vi "GEA2 Commands Dryer CMD.vi"() -> (2 "CMD Array":u8[](array[numeric])=[115, 0] format="%02x")   [LabVIEW 2016]
doc: "Given the command array, this VI will look up the associated Hex numaric and output that value"
panel:
  in  "Commands":cluster{"String":string, "CMD Array":u8[]}[](array[cluster])=[{"String"="CMD_Eval_Mode_Entry_CC1", "CMD Array"=[112, 1]}, {"String"="CMD_Eval_Mode_Entry_CC2", "CMD Array"=[112, 2]}, {"String"="CMD_Eval_Mode_Continue", "CMD Array"=[113]}, {"String"="CMD_Send_DIAG_Info", "CMD Array"=[114]}, {"String"="CMD_Enable_Debug_Log ", "CMD Array"=[115, 1]}, {"String"="CMD_Disable_Debug_Log ", "CMD Array"=[115, 0]}, {"String"="CMD_Send_Log_Data", "CMD Array"=[116]}, {"String"="CMD_Stop", "CMD Array"=[118]}, {"String"="RQST_Version", "CMD Array"=[1]}] {"CMD Array" format="%02x"}
  out "Data Array":string[][](array[string])=[["CMD_Eval_Mode_Entry_CC1", "0x70", "0x01"], ["CMD_Eval_Mode_Entry_CC2", "0x70", "0x02"], ["CMD_Eval_Mode_Continue", "0x71", "N/A"], ["CMD_Send_DIAG_Info", "0x72", "N/A"], ["CMD_Enable_Debug_Log ", "0x73", "0x01"], ["CMD_Disable_Debug_Log ", "0x73", "0x00"], ["CMD_Send_Log_Data", "0x74", "N/A"]]
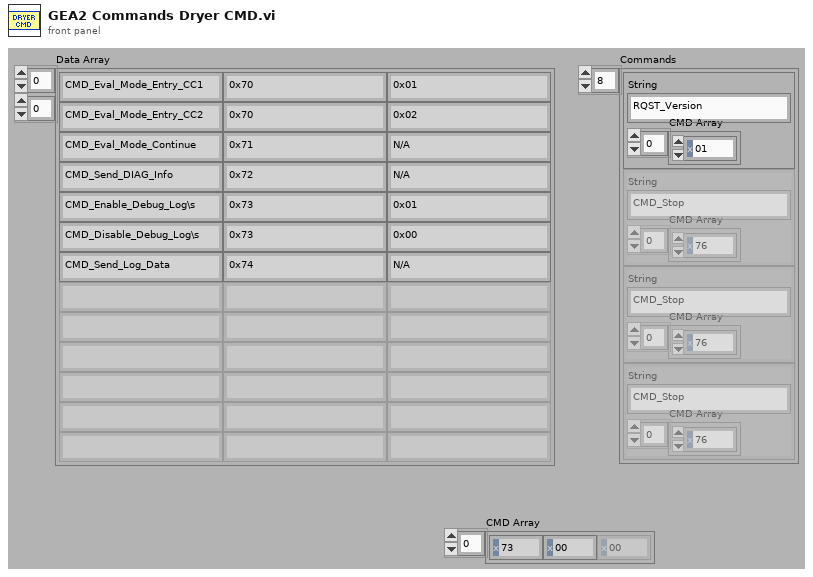
[diagram p1: front panel]
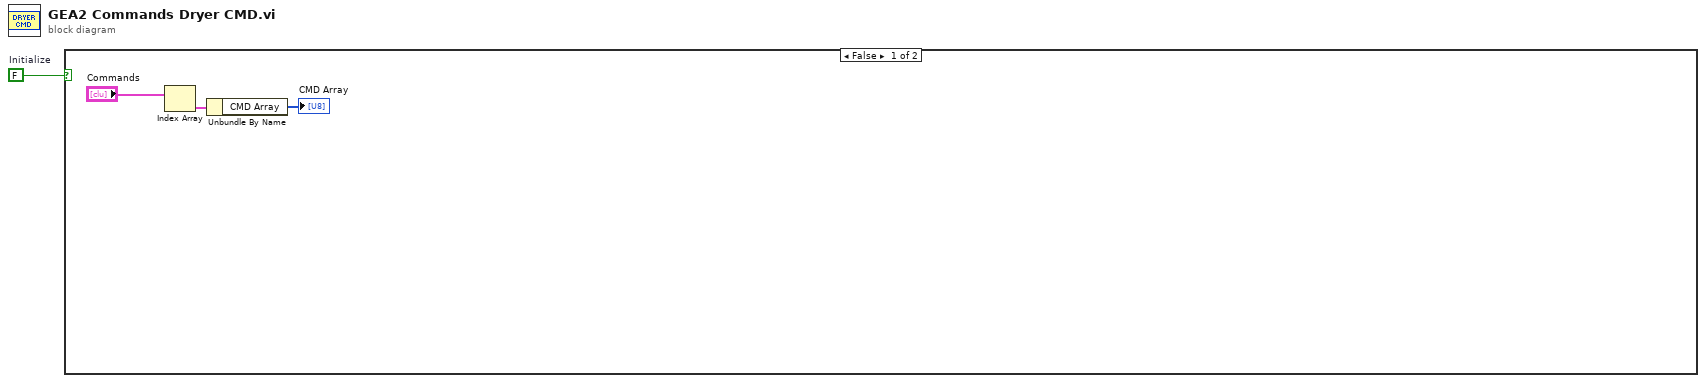
[diagram p0: block diagram]
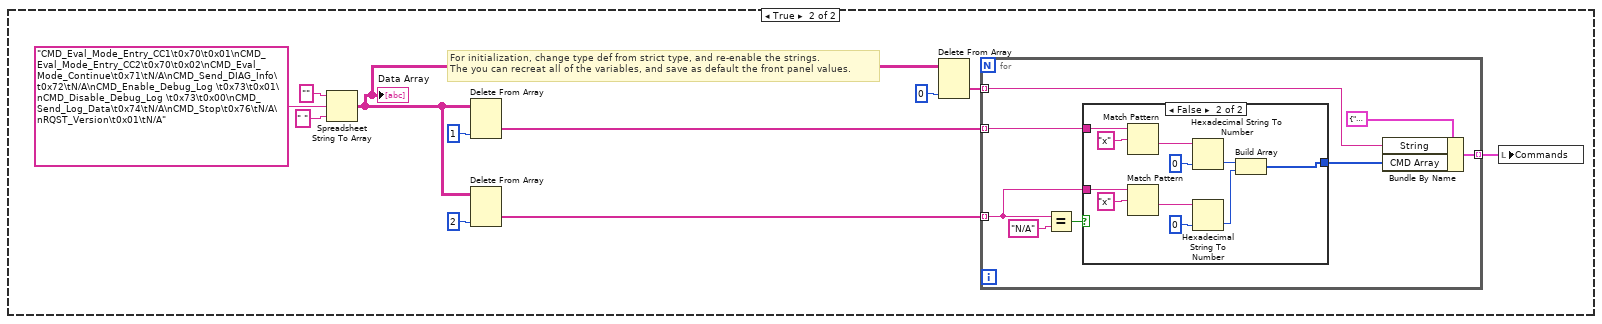
[diagram p2: hidden frame]
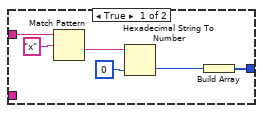
[diagram p3: hidden frame]
diagram:
  w1 = FALSE  # Initialize
  n1 = case shown="False" w1 {
    frame False {
      n2 = Index Array(array="Commands") -> (element=w3:cluster{"String":string, "CMD Array":u8[]})  [unwired: 1 in]
      n3 = Unbundle By Name(w3) -> ("CMD Array"=→"CMD Array":u8[])
    }
    frame True {
      # "For initialization, change type def from strict type, and re-enable the strings.\nThe you can recreat all of the variables, and save as default the front panel values."
      n4 = Spreadsheet String To Array(format string="", spreadsheet string="CMD_Eval_Mode_Entry_CC1\t0x70\t0x01\nCMD_Eval_Mode_Entry_CC2\t0x70\t0x02\nCMD_Eval_Mode_Continue\t0x71\tN/A\nCMD_Send_DIAG_Info\t0x72\tN/A\nCMD_Enable_Debug_Log \t0x73\t0x01\nCMD_Disable_Debug_Log \t0x73\t0x00\nCMD_Send_Log_Data\t0x74\tN/A\nCMD_Stop\t0x76\tN/A\nRQST_Version\t0x01\tN/A", array type (2D Dbl)=" " ("delimiter (Tab)")) -> (array=w8:string[][])  [unwired: 1 in]
      "Data Array" <- w8
      n5 = Delete From Array(array=w8, index (col)=1 ("disabled index (col)")) -> (deleted portion=w10:string[])  [unwired: 2 in, 1 out]
      n6 = Delete From Array(array=w8, index (col)=2 ("disabled index (col)")) -> (deleted portion=w7:string[])  [unwired: 2 in, 1 out]
      n7 = Delete From Array(array=w8, index (col)=0 ("disabled index (col)")) -> (deleted portion=w5:string[])  [unwired: 2 in, 1 out]
      n8 = for {
        tunnel: w5 -> [w22] mode=indexing
        tunnel: w10 -> [w21] mode=indexing
        tunnel: [w20] -> w6 mode=indexing
        tunnel: w7 -> [w16] mode=indexing
        n9 = Equal?(x=w16, y="N/A") -> (x = y?=w17:bool)
        n10 = case shown="False" w17 {
          tunnel: w21 -> [w29 w40]
          tunnel: [w24 w36] -> w19
          tunnel: w16 -> [_ w34]
          frame True {
            n11 = Match Pattern(string=w29, regular expression="x") -> (after substring=w27:string)  [unwired: 1 in, 3 out]
            n12 = Hexadecimal String To Number(string=w27, default (0uL)=u8 0 ("default (0 U32)")) -> (number=w25:u8)  [unwired: 1 in, 1 out]
            n13 = Build Array(w25) -> (w24:u8[])
          }
          frame False {
            n14 = Match Pattern(string=w40, regular expression="x") -> (after substring=w38:string)  [unwired: 1 in, 3 out]
            n15 = Match Pattern(string=w34, regular expression="x") -> (after substring=w31:string)  [unwired: 1 in, 3 out]
            n16 = Hexadecimal String To Number(string=w38, default (0uL)=u8 0 ("default (0 U32)")) -> (number=w37:u8)  [unwired: 1 in, 1 out]
            n17 = Hexadecimal String To Number(string=w31, default (0uL)=u8 0 ("default (0 U32)")) -> (number=w30:u8)  [unwired: 1 in, 1 out]
            n18 = Build Array(w37, w30) -> (w36:u8[])
          }
        }
        n19 = Bundle By Name(cluster=cluster{"String":string, "CMD Array":u8[]} {"String"="100 Hz", "CMD Array"=[]}, "String"=w22, "CMD Array"=w19) -> (w20:cluster{"String":string, "CMD Array":u8[]})
      }
      n20 = local write "Commands"(w6) -> ()
    }
  }
